vi "q1 string conditional concatenation.vi"() -> ()   [LabVIEW 2025]
panel:
  out "OUTPUT":string
  out "LENGTH":i32
  in  "N":dbl
  in  "B":string
  in  "A":string
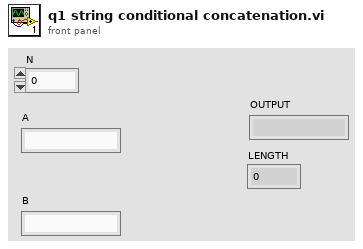
[diagram p1: front panel]
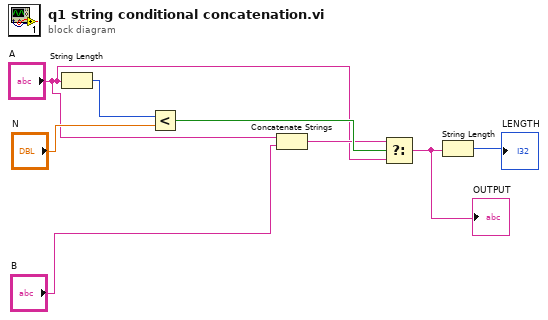
[diagram p0: block diagram]
diagram:
  n1 = String Length(string="A") -> (length=w8:i32)
  n2 = Less?(x=w8, y="N") -> (x < y?=w5:bool)
  n3 = Concatenate Strings("A", "B") -> (w4:string)
  n4 = Select(t=w4, s=w5, f="A") -> (s? t:f=w1:string)
  "OUTPUT" <- w1
  n5 = String Length(string=w1) -> (length=→"LENGTH":i32)
